vi "o3 Serial Comms Test.vi"() -> ()   [LabVIEW 2014]
uses:
  <vilib>/Platform/TimedLoop/XDataNode/timing_clust.ctl
  <vilib>/Platform/TimedLoop/XDataNode/nitl_modes.ctl
  <vilib>/Platform/TimedLoop/XDataNode/wakeup.ctl
  <vilib>/Utility/error.llb/whitespace.ctl
  <vilib>/Instr/_visa.llb/VISA Configure Serial Port (Instr).vi
  <vilib>/platform/TimedLoop/XDataNode/XDataNode.xnode
  <vilib>/Platform/TimedLoop/XDataNode/XDNodeRunTimeDep.lvlib
panel:
  in  "stop 2":bool
  out "Internal packet":string[](array[string])
  out "Data String":string
  out "Read Error Counter\nfrom process loop":i32
  out "Scan from String Error Counter\nfrom process loop":i32
  out "Data Array":string[](array[string])
  out "Data Processing":bool
  out "Serial Visa Error":errorcluster
  out "output 1":string
  out "error out 2":errorcluster
  out "Data In Array":string[](array[string])
  out "Number of Send & Read Error\nfrom Acquire Loop":i32
  out "Command In":string
  out "RAW DATA":string
  in  "ID 2":string="‚"
  in  "stop":bool
  in  "Command Input":string
  in  "VISA resource name 2":refnum<visa-resource-name>="ASRL6::INSTR"
  out "error out":errorcluster
  in  "Wait Time(mSec)":u32=330 caption="Count(mSec)"
  out "Loop counter":i32
  out "Max Acq Time":u32
  out "Write & Read Time (msec)":u32(graph)
  out "Running?":bool
  out "String":string
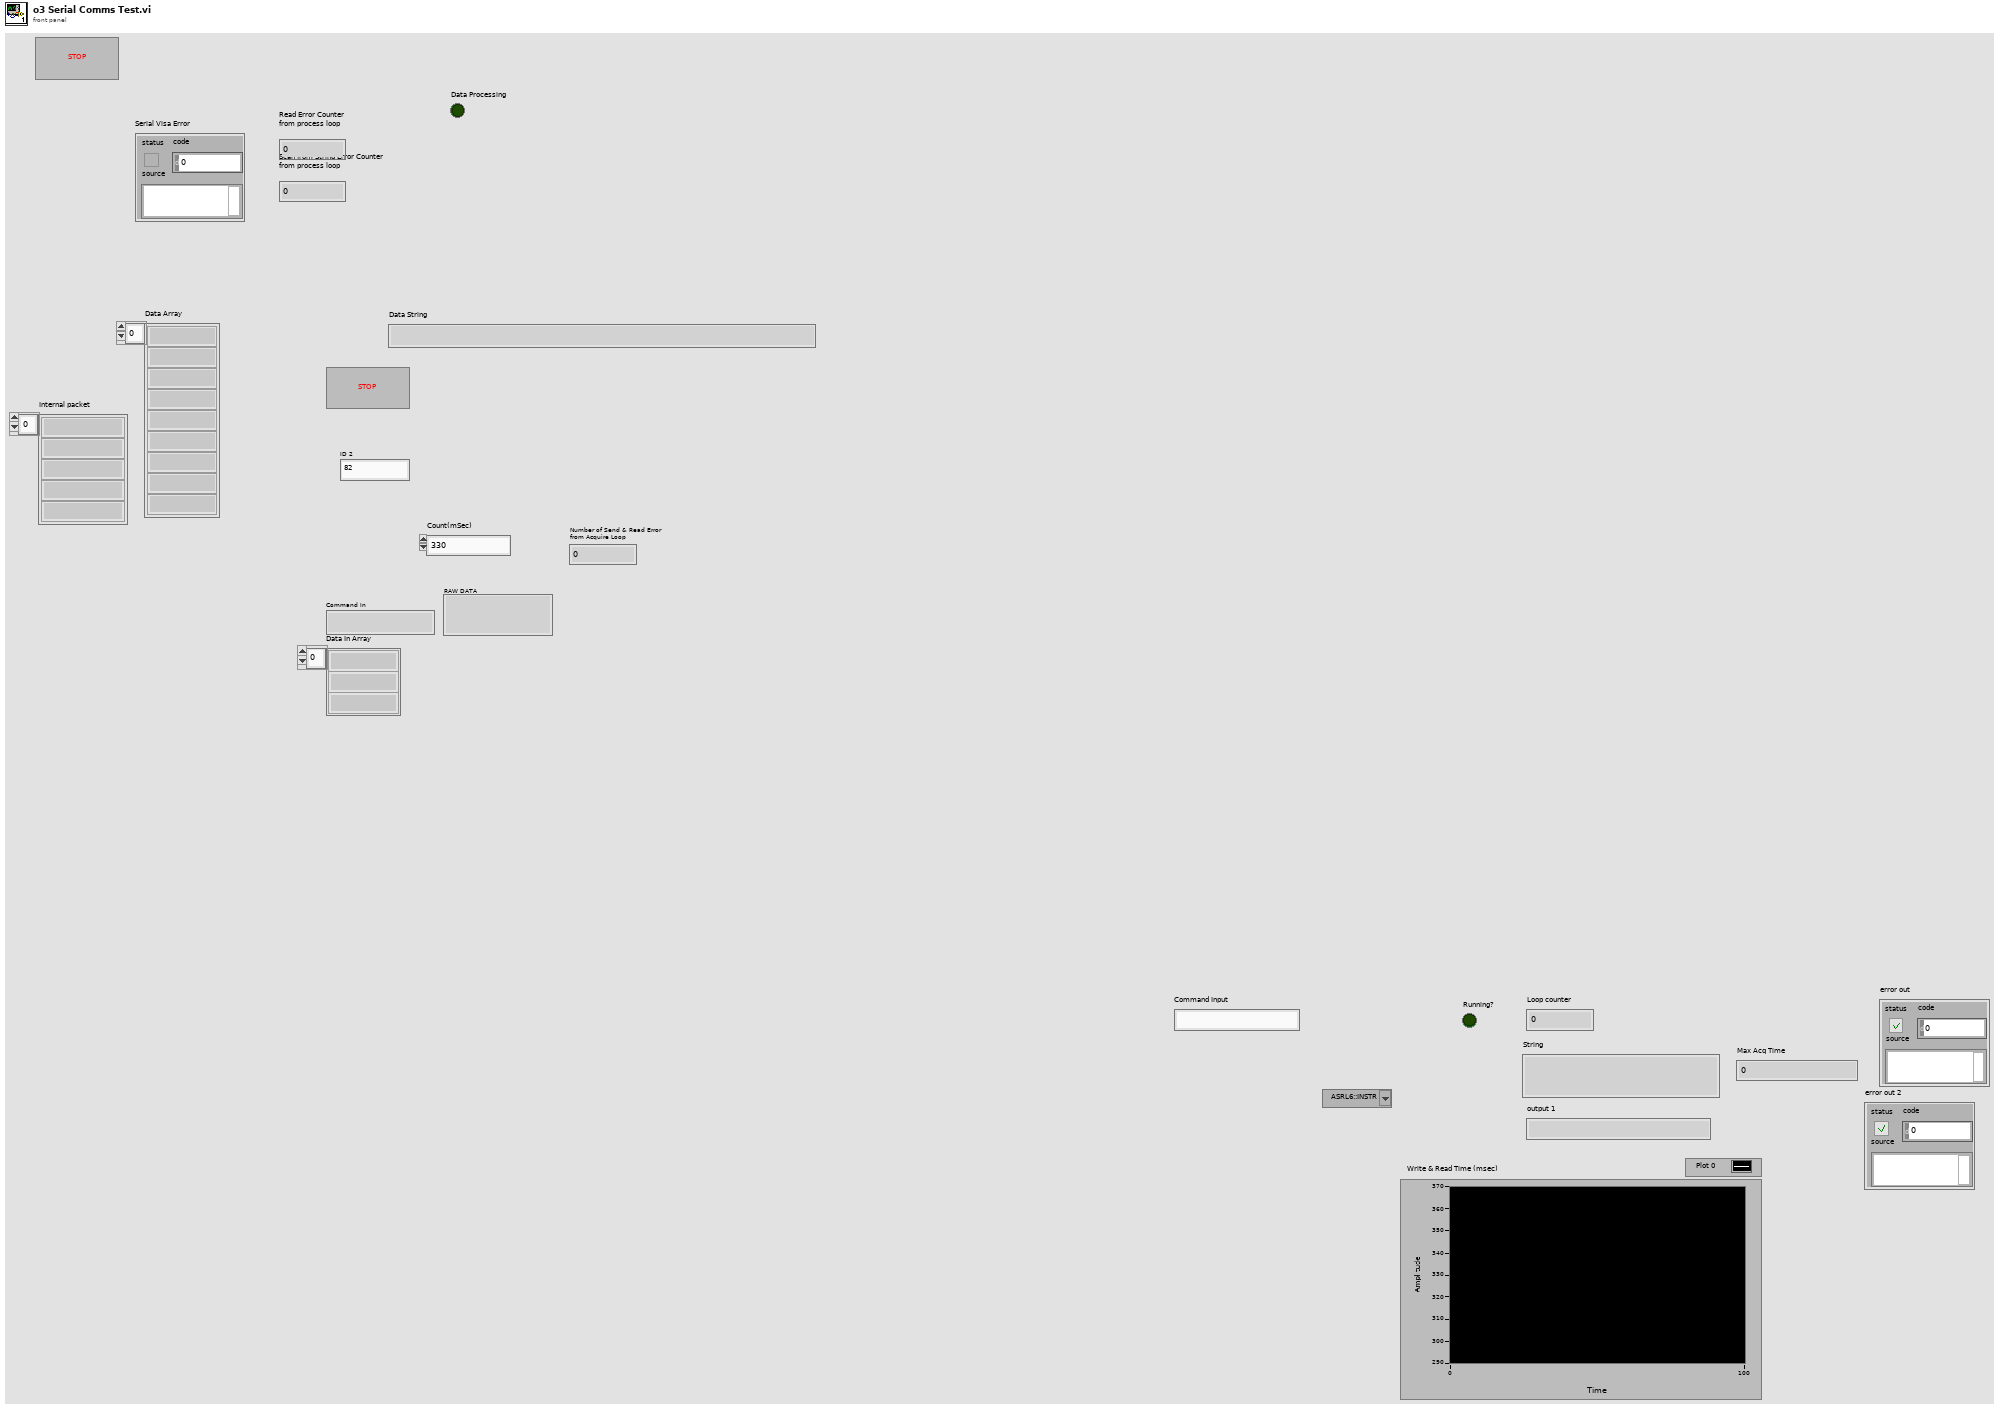
[diagram p1: front panel]
types:
  T1 = typedef "XDNodeRunTimeDep.lvlib/timing_clust.ctl" = cluster{"Expected End [f-1]":u64, "Actual End [f-1]":u64, "Finished Late? [f-1]":bool, "Expected End [i-1]":u64, "Actual End [i-1]":u64, "Finished Late? [i-1]":bool, "Expected Start [i]":u64, "Actual Start [i]":u64, "Expected Start [f]":u64, "Actual Start [f]":u64, "Source Name":string, "Structure Name":string, "Period":i64, "Deadline":i64, "Offset":i64, "Start":i64, "Priority":i32, "Timeout":i32, "Mode":T2, "Wakeup Reason":T3, "Error":errorcluster, "Source Type":string, "Secondary Source Type":string, "Global End Time":u64, "Global Start Time":u64, "Frame Duration":u64, "Iteration Duration":u64, "Assigned CPU":i32, "I/O Scan Engine Mode":u32}
  T2 = typedef "XDNodeRunTimeDep.lvlib/nitl_modes.ctl" = enum32{"No Change", "Process missed periods, maintain original phase", "Discard missed periods, maintain original phase", "Process missed periods, ignore original phase", "Discard missed periods, ignore original phase"}
  T3 = typedef "XDNodeRunTimeDep.lvlib/wakeup.ctl" = enum32{"Normal", "Aborted", "Asynchronous wakeup", "Timing source error", "Timed loop error", "Timeout"}
  T4 = typedef "whitespace.ctl" = u16
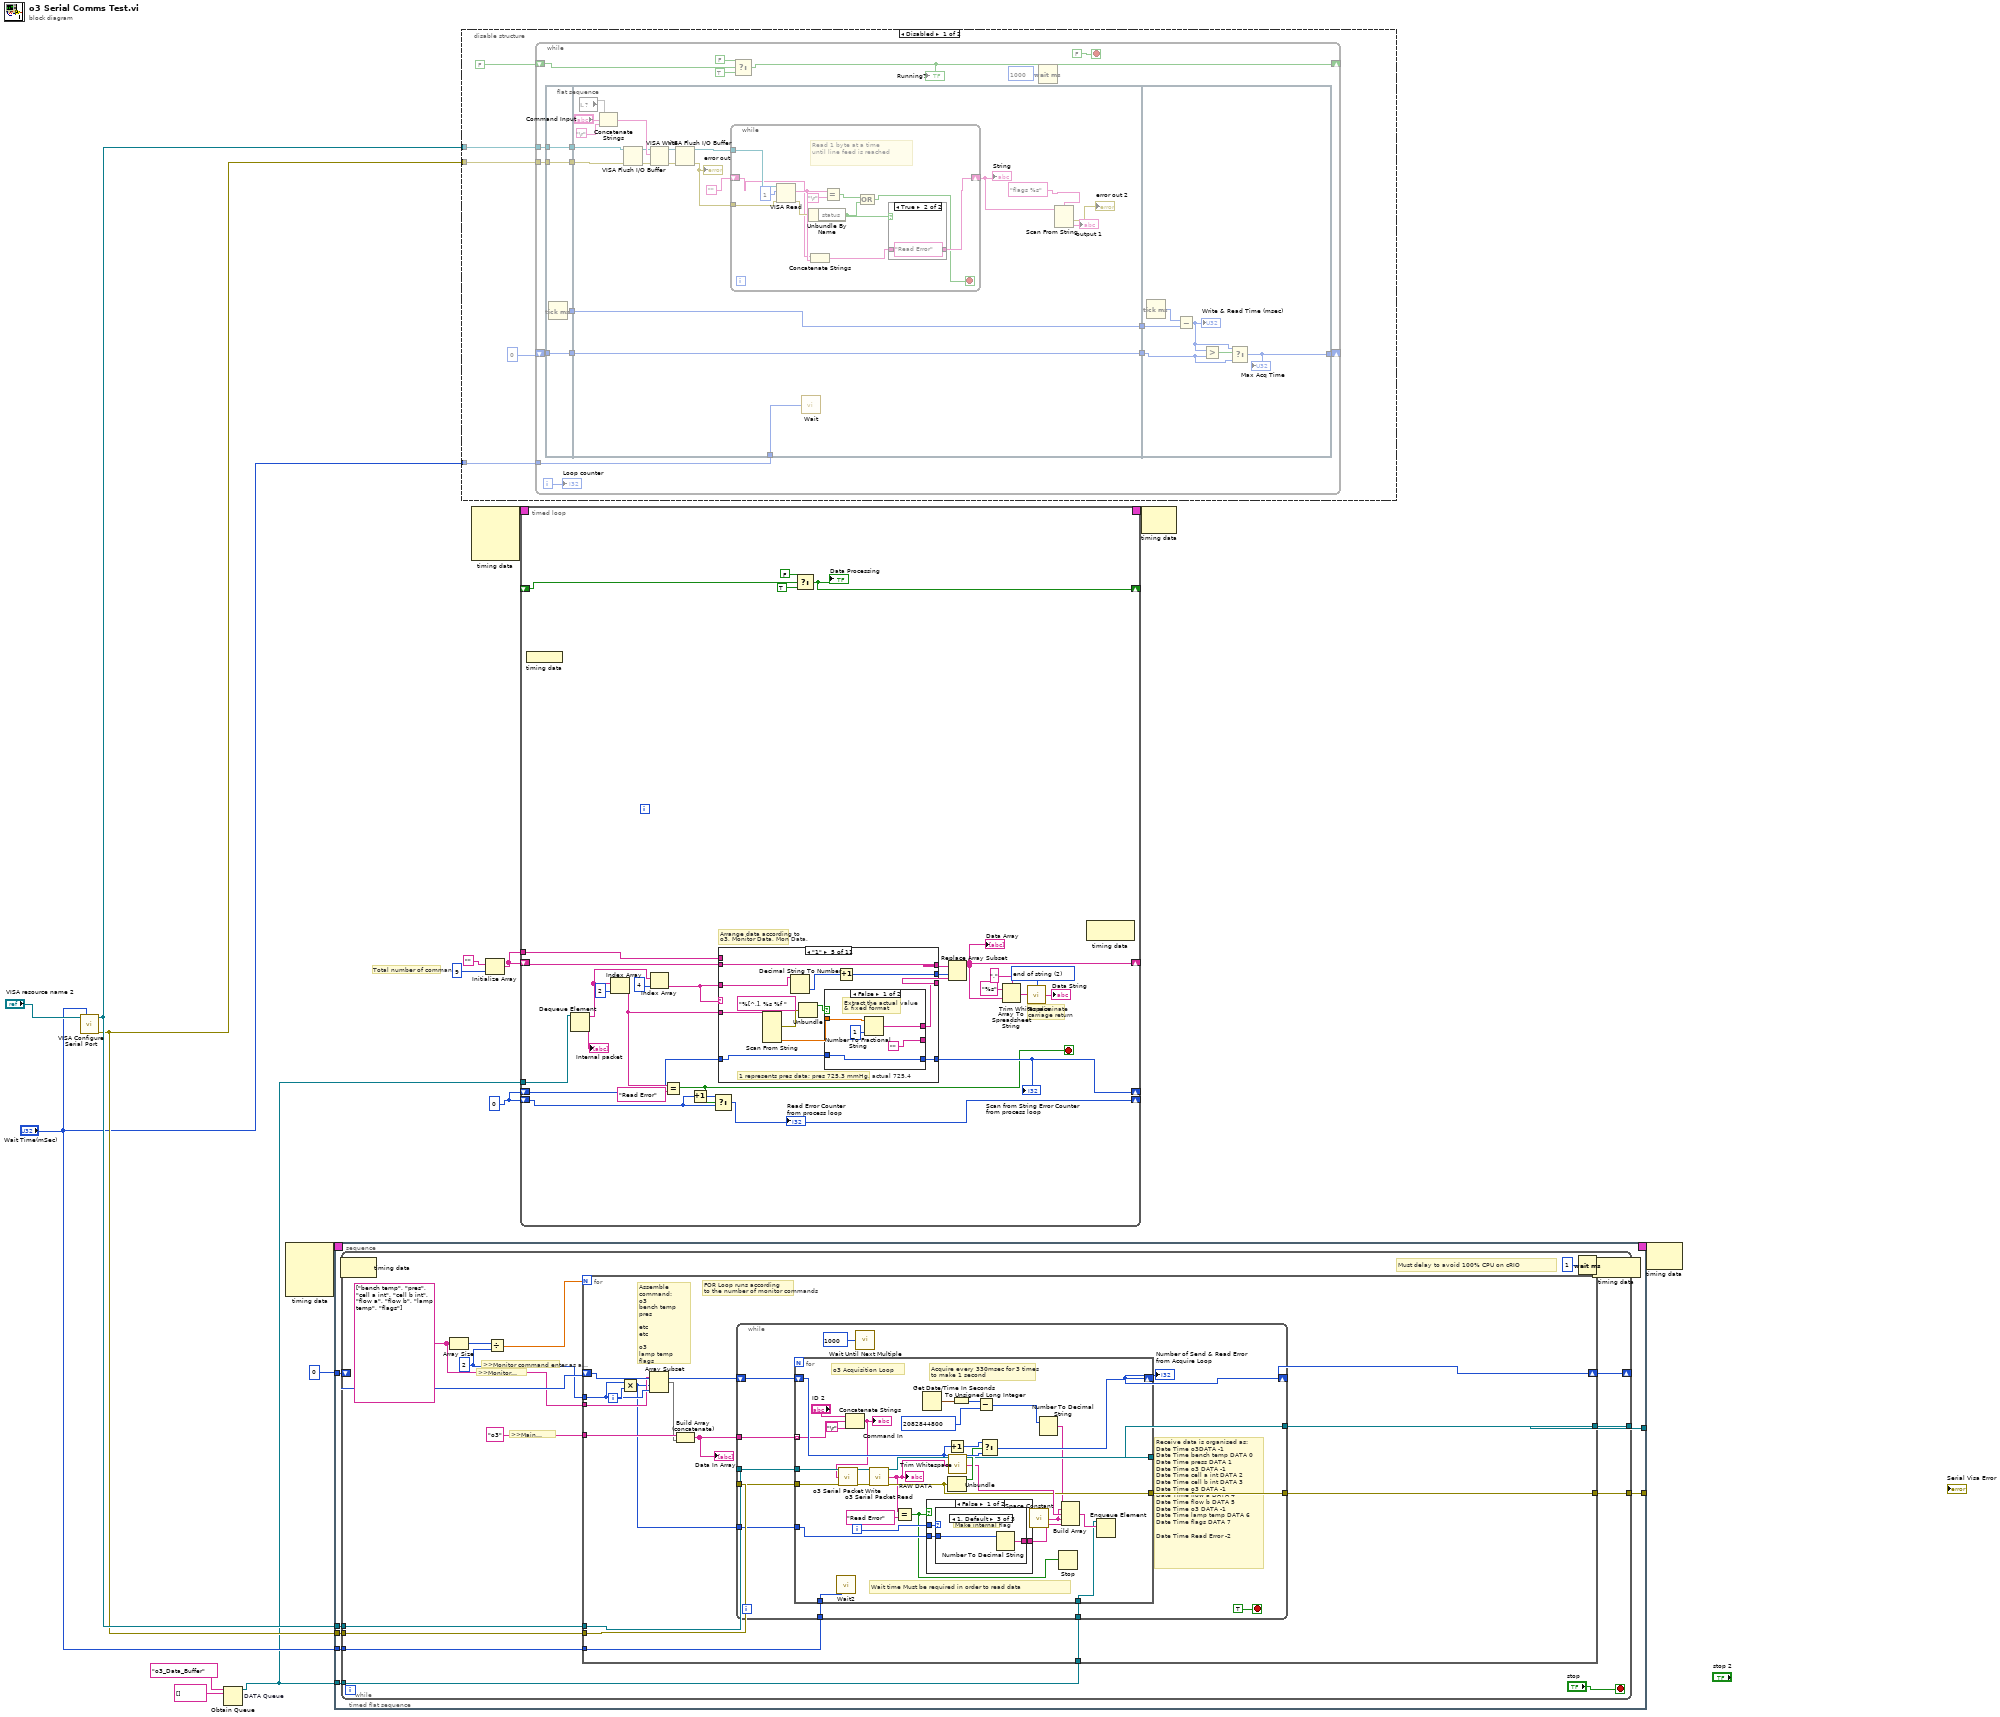
[diagram p0: block diagram]
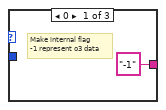
[diagram p2: hidden frame]
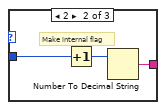
[diagram p3: hidden frame]
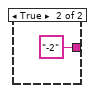
[diagram p4: hidden frame]
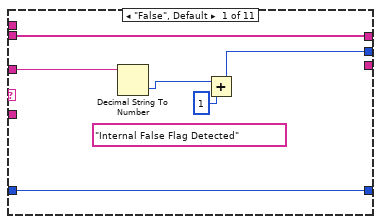
[diagram p7: hidden frame]
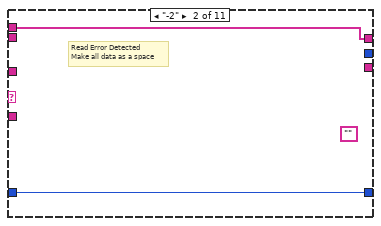
[diagram p8: hidden frame]
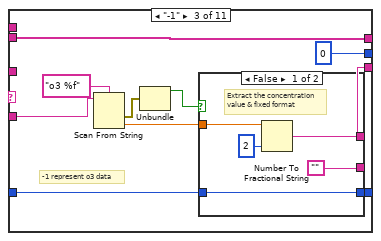
[diagram p9: hidden frame]
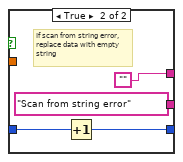
[diagram p10: hidden frame]
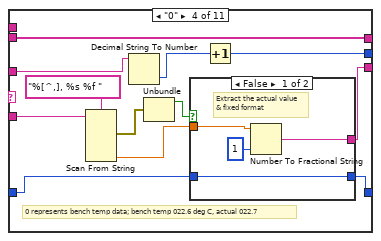
[diagram p11: hidden frame]
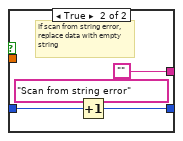
[diagram p12: hidden frame]
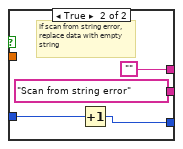
[diagram p13: hidden frame]
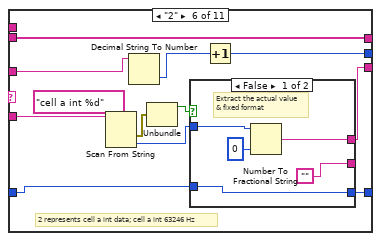
[diagram p14: hidden frame]
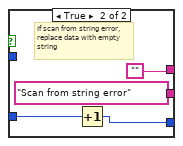
[diagram p15: hidden frame]
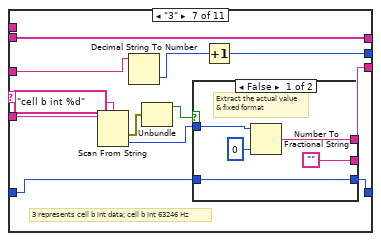
[diagram p16: hidden frame]
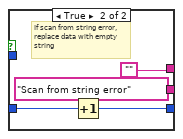
[diagram p17: hidden frame]
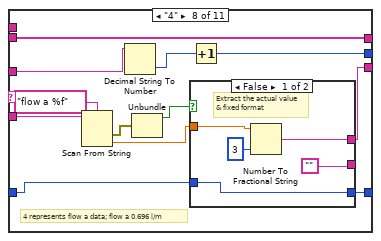
[diagram p18: hidden frame]
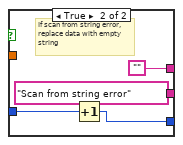
[diagram p19: hidden frame]
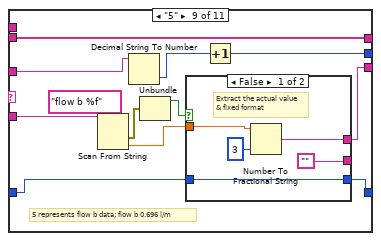
[diagram p20: hidden frame]
diagram:
  w4 = 0
  # "Total number of commands"
  n1 = call-poly "VISA Configure Serial Port"("VISA resource name"="VISA resource name 2", "timeout (10sec)"="Wait Time(mSec)") -> ("VISA resource name out"=w15:refnum<visa-resource-name>, "error out"=w14:errorcluster)  [unwired: 12 in]
  n2 = Obtain Queue "DATA Queue"(name (unnamed)="o3_Data_Buffer", element data type=string[] []) -> (queue out=w5:refnum<queue>)  [unwired: 3 in, 2 out]
  n3 = node-c288() -> (w8:T1)  [unwired: 4 in]
  n4 = timed-sequence {
    timing: w8 -> [_]
    timing-out: [_] -> w7
    tunnel: [w23] -> _
    tunnel: [w22] -> _
    tunnel: 0 -> [w21]
    tunnel: w14 -> [w20]
    tunnel: w15 -> [w19]
    tunnel: "Wait Time(mSec)" -> [w18]
    tunnel: w5 -> [w17]
    n5 = timed-flat-sequence {
      tunnel: [w30] -> w23
      tunnel: [w29] -> w22
      tunnel: w21 -> [w28]
      tunnel: w20 -> [w27]
      tunnel: w19 -> [w26]
      tunnel: w18 -> [w25]
      tunnel: w17 -> [w24]
      n6 = node-c288() -> ()  [unwired: 1 in, 1 out]
      n7 = while {
        tunnel: [w35] -> w30
        tunnel: w26 -> [w45]
        tunnel: w27 -> [w44]
        tunnel: [w43] -> w29
        shift-right: [w41] -> _
        shift-left: w28 -> [w42]
        tunnel: w25 -> [w33]
        tunnel: w24 -> [w31]
        stop <- "stop" stop-if-true
        w36 = 2
        w38 = string[] ["bench temp", "pres", "cell a int", "cell b int", "flow a", "flow b", "lamp temp", "flags"]
        # "Must delay to avoid 100% CPU on cRIO"
        # ">>Monitor command enter as a pair>>"
        # ">>Main commands>>"
        # ">>Monitor Command>>"
        n8 = Array Size(array=w38) -> (size(s)=w39:i32)
        n9 = Divide(x=w39, y=w36) -> (x/y=w37:dbl)
        n10 = for {
          N: w37 -> [_]
          tunnel: w45 -> [w54]
          tunnel: w44 -> [w53]
          tunnel: [w60] -> w35
          shift-right: [w58] -> w41
          shift-left: w42 -> [w59]
          tunnel: [w57] -> w43
          tunnel: w38 -> [w50]
          tunnel: "o3" -> [w55]
          tunnel: w36 -> [w51]
          tunnel: w33 -> [w47]
          tunnel: w31 -> [w46]
          i -> [w52]
          # "FOR Loop runs according\nto the number of monitor commands"
          # "Assemble command:\no3\nbench temp\npres\n\netc\netc\n\no3\nlamp temp\nflags"
          n11 = Multiply(x=w51, y=w52) -> (x*y=w48:i32)
          n12 = Array Subset(array=w50, index=w48, length=w51) -> (w49:string[])
          n13 = Build Array (concatenate)(w55, w49) -> (w56:string[])
          "Data In Array" <- w56
          n14 = while {
            tunnel: [w72] -> w60
            tunnel: w56 -> [w70]
            tunnel: [w68] -> w57
            tunnel: w53 -> [w67]
            tunnel: w54 -> [w66]
            tunnel: w48 -> [w65]
            shift-right: [w69] -> w58
            shift-left: w59 -> [w71]
            tunnel: w47 -> [w62]
            tunnel: w46 -> [w61]
            stop <- TRUE stop-if-true
            # "Receive data is organised as:\nDate Time o3DATA -1\nDate Time bench temp DATA 0\nDate Time press DATA 1\nDate Time o3 DATA -1\nDate Time cell a int DATA 2\nDate Time cell b int DATA 3\nDate Time o3 DATA -1\nDate Time flow a DATA 4\nDate Time flow b DATA 5\nDate Time o3 DATA -1\nDate Time lamp temp DATA 6\nDate Time flags DATA 7\n\nDate Time Read Error -2"
            n15 = for {
              tunnel: w67 -> [w90]
              tunnel: [w91] -> w72
              tunnel: w70 -> [w88] mode=indexing
              tunnel: [w92] -> w68
              tunnel: w66 -> [w93]
              tunnel: w65 -> [w87]
              shift-right: [w101] -> w69
              shift-left: w71 -> [w102]
              tunnel: w62 -> [w78]
              tunnel: w61 -> [w74]
              i -> [w82]
              # "Wait time Must be required in order to read data"
              # "Acquire every 330msec for 3 times\nto make 1 second"
              # "o3 Acquisition Loop"
              n16 = call "Wait2"("Count(mSec)"=w78) -> ()  [unwired: 1 out]
              n17 = Concatenate Strings("ID 2", w88, "\r") -> (w86:string)
              "Command In" <- w86
              n18 = call "o3 Serial Packet Write.vi"("VISA resource name In"=w93, "Data in"=w86, "error in (no error)"=w90) -> ("VISA resource name Out"=w95:refnum<visa-resource-name>, "error out"=w94:errorcluster)  [unwired: 11 in]
              n19 = call "o3 Serial Packet Read.vi"("VISA resource In"=w95, "error in"=w94) -> ("VISA resource Out"=w92:refnum<visa-resource-name>, "Data Out"=w84:string, "error out"=w91:errorcluster)  [unwired: 11 in]
              "RAW DATA" <- w84
              n20 = Equal?(x=w84, y="Read Error") -> (x = y?=w73:bool)
              n21 = Get Date/Time In Seconds() -> (seconds since 1Jan1904=w77:timestamp)
              n22 = case shown="False" w73 {
                tunnel: [w105 "-2"] -> w96
                tunnel: w82 -> [w104 _]
                tunnel: w87 -> [w103 _]
                frame False {
                  n23 = case shown="1, Default" w104 {
                    tunnel: ["-1" w109 w111] -> w105
                    tunnel: w103 -> [_ w107 w110]
                    frame 0 {
                      # "Make internal flag\n-1 represent o3 data"
                    }
                    frame 2 {
                      # "Make internal flag"
                      n24 = Increment(x=w107) -> (x+1=w108:i32)
                      n25 = Number To Decimal String(number=w108) -> (decimal integer string=w109:string)  [unwired: 1 in]
                    }
                    frame 1, Default {
                      # "Make internal flag"
                      n26 = Number To Decimal String(number=w110) -> (decimal integer string=w111:string)  [unwired: 1 in]
                    }
                  }
                }
                frame True {
                }
              }
              n27 = Increment(x=w102) -> (x+1=w98:i32)
              n28 = Unbundle(w91) -> ("status"=w99:bool)  [unwired: 2 out]
              n29 = call <vilib>:"Trim Whitespace.vi"("string"=w84) -> ("trimmed string"=w97:string)  [unwired: 1 in]
              n30 = To Unsigned Long Integer(number=w77) -> (unsigned 32bit integer=w81:u32)
              n31 = Subtract(x=w81, y=u32 2082844800) -> (x-y=w76:u32)
              n32 = Select(t=w98, s=w99, f=w102) -> (s? t:f=w101:i32)
              n33 = call <vilib>:"Space Constant.vi"() -> ("String"=w85:string)
              n34 = Number To Decimal String(number=w76) -> (decimal integer string=w79:string)  [unwired: 1 in]
              n35 = Stop(stop? (T)=w73) -> ()
              n36 = Build Array(w79, w85, w97, w85, w96) -> (w75:string[])
              n37 = Enqueue Element(queue=w74, element=w75) -> ()  [unwired: 2 in, 3 out]
            }
            "Number of Send & Read Error\nfrom Acquire Loop" <- w69
            n38 = call "Wait Until Next Multiple"("Count(mSec)"=u32 1000) -> ()  [unwired: 1 out]
          }
        }
        n39 = Wait (ms)(milliseconds to wait=u32 1) -> ()  [unwired: 1 out]
      }
      n40 = node-c288() -> ()  [unwired: 1 in, 1 out]
    }
  }
  n41 = disable-structure shown="Disabled" {
    disable-tunnel: w15 -> [w119 _]
    disable-tunnel: w14 -> [w118 _]
    disable-tunnel: "Wait Time(mSec)" -> [w117 _]
    frame Disabled {
      n42 = while {
        tunnel: w119 -> [w137]
        tunnel: w118 -> [w136]
        shift-right: [w131] -> _
        shift-left: FALSE -> [w134]
        shift-right: [w122] -> _
        shift-left: u32 0 -> [w124]
        tunnel: w117 -> [w120]
        i -> [w121]
        stop <- FALSE stop-if-true
        n43 = flat-sequence {
          tunnel: w136 -> [w140]
          tunnel: w137 -> [w141]
          tunnel: [w141] -> w129
          tunnel: [w140] -> w128
          tunnel: [w139] -> w127
          tunnel: [w138] -> w125
          tunnel: w124 -> [w138]
          tunnel: w129 -> [w155]
          tunnel: w128 -> [w154]
          tunnel: w127 -> [w149]
          tunnel: [w149] -> w126
          tunnel: w125 -> [w148]
          tunnel: [w148] -> w123
          tunnel: w120 -> [w147]
          tunnel: w126 -> [w180]
          tunnel: w123 -> [w177]
          tunnel: [w176] -> w122
          frame #0 {
            n44 = Tick Count (ms)() -> (millisecond timer value=w139:u32)
          }
          frame #1 {
            n45 = local read item#-1() -> (w161)
            n46 = Concatenate Strings(w161, "Command Input", "\r") -> (w157:string)
            n47 = VISA Flush I/O Buffer(VISA resource name=w155, error in (no error)=w154) -> (VISA resource name out=w156:refnum<visa-resource-name>, error out=w159:errorcluster)  [unwired: 1 in]
            n48 = VISA Write(VISA resource name=w156, write buffer=w157, error in (no error)=w159) -> (VISA resource name out=w153:refnum<visa-resource-name>, error out=w160:errorcluster)  [unwired: 1 out]
            n49 = VISA Flush I/O Buffer(VISA resource name=w153, error in (no error)=w160) -> (VISA resource name out=w151:refnum<visa-resource-name>, error out=w150:errorcluster)  [unwired: 1 in]
            "error out" <- w150
            n50 = while {
              shift-right: [w164] -> w144
              shift-left: "" -> [w165]
              tunnel: w151 -> [w166]
              tunnel: w150 -> [w162]
              stop <- w163 stop-if-true
              # "Read 1 byte at a time \nuntil line feed is reached"
              n51 = VISA Read(VISA resource name=w166, byte count=u32 1, error in (no error)=w162) -> (read buffer=w173:string, error out=w170:errorcluster)  [unwired: 2 out]
              n52 = Unbundle By Name(w170) -> ("status"=w168:bool)
              n53 = Concatenate Strings(w165, w173) -> (w169:string)
              n54 = Equal?(x=w173, y="\r") -> (x = y?=w167:bool)
              n55 = Compound Arithmetic op=OR(w167, w168) -> (w163:bool)
              n56 = case shown="True" w168 {
                tunnel: w169 -> [w174 _]
                tunnel: [w174 "Read Error"] -> w164
                frame False {
                }
                frame True {
                }
              }
            }
            "String" <- w144
            n57 = call "Wait"("Count(mSec)"=w147) -> ()  [unwired: 1 out]
            n58 = Scan From String(format string="flags %s", input string=w144) -> (error out=→"error out 2":errorcluster, output 1=→"output 1":string)  [unwired: 3 in, 2 out]
          }
          frame #2 {
            n59 = Tick Count (ms)() -> (millisecond timer value=w181:u32)
            n60 = Subtract(x=w181, y=w180) -> (x-y=w178:u32)
            "Write & Read Time (msec)" <- w178
            n61 = Greater?(x=w178, y=w177) -> (0:w179:bool)
            n62 = Select(t=w178, s=w179, f=w177) -> (s? t:f=w176:u32)
            "Max Acq Time" <- w176
          }
        }
        n63 = Select(t=FALSE, s=w134, f=TRUE) -> (s? t:f=w131:bool)
        "Running?" <- w131
        n64 = Wait (ms)(milliseconds to wait=u32 1000) -> ()  [unwired: 1 out]
        "Loop counter" <- w121
      }
    }
    frame Enabled {
    }
  }
  n65 = node-c288() -> (w12:T1)  [unwired: 4 in]
  n66 = Initialize Array("", 9) -> (w1:string[])
  n67 = timed-loop {
    timing: w12 -> [_]
    timing-out: [_] -> w11
    tunnel: w5 -> [w209]
    shift-right: [w189] -> _
    shift-left: w1 -> [w206]
    shift-right: [w195] -> _
    shift-left: w4 -> [w192]
    tunnel: w1 -> [w194]
    shift-right: [w190] -> _
    shift-left: w4 -> [w191]
    shift-right: [w184] -> _
    shift-left: _ -> [w186]
    stop <- w182 stop-if-true
    w199 = T4 2 items=["both", "start of string", "end of string"] ("location (both)")
    # "Arrange data according to\no3, Monitor Data, Mon Data,"
    # "To eliminate\ncarriage return"
    n68 = node-c288() -> ()  [unwired: 1 in]
    n69 = Dequeue Element(queue=w209) -> (element=w187:string[])  [unwired: 2 in, 3 out]
    "Internal packet" <- w187
    n70 = Index Array(array=w187, index=2) -> (element=w197:string)
    n71 = Index Array(array=w187, index=4) -> (element=w205:string)
    n72 = Equal?(x=w197, y="Read Error") -> (x = y?=w182:bool)
    n73 = Increment(x=w192) -> (x+1=w193:i32)
    n74 = Select(t=w193, s=w182, f=w192) -> (s? t:f=w195:i32)
    "Read Error Counter\nfrom process loop" <- w195
    n75 = case shown="\"1\"" w205 {
      tunnel: w205 -> [w214 _ _ w247 w266 w287 w308 w329 w350 w371 w392]
      tunnel: w206 -> [w215 _ w227 w248 w267 w288 w309 w330 w351 w372 w393]
      tunnel: w197 -> [_ _ w224 w243 w262 w284 w305 w326 w347 w368 w389]
      tunnel: [w215 w217 w227 w248 w267 w288 w309 w330 w351 w372 w393] -> w204
      tunnel: [w212 _ 0 ("index") w245 w264 w285 w306 w327 w348 w369 w390] -> w203
      tunnel: [_ _ w222 w241 w260 w283 w304 w325 w346 w367 w384] -> w202
      tunnel: w194 -> [_ w217 _ _ _ _ _ _ _ _ _]
      tunnel: w191 -> [w210 w216 w219 w238 w257 w278 w299 w320 w341 w362 w383]
      tunnel: [w210 w216 w218 w237 w256 w277 w298 w319 w340 w361 w382] -> w190
      frame "False", Default {
        (unwired) "Internal False Flag Detected"
        n76 = Decimal String To Number(string=w214) -> (number=w211:i32)  [unwired: 2 in, 1 out]
        n77 = Add(x=w211, y=1) -> (x+y=w212:i32)
      }
      frame "-2" {
        (unwired) ""
        # "Read Error Detected\nMake all data as a space"
      }
      frame "-1" {
        # "-1 represent o3 data"
        n78 = Scan From String(format string="o3 %f", input string=w224) -> (error out=w221:errorcluster, output 1=w223:dbl)  [unwired: 3 in, 2 out]
        n79 = Unbundle(w221) -> ("status"=w220:bool)  [unwired: 2 out]
        n80 = case shown="False" w220 {
          tunnel: w223 -> [w232 _]
          tunnel: [w231 ""] -> w222
          tunnel: w219 -> [w230 w235]
          tunnel: [w230 w234] -> w218
          tunnel: ["" "Scan from string error"] -> _
          frame False {
            # "Extract the concentration\nvalue & fixed format"
            n81 = Number To Fractional String(number=w232, precision (6)=i16 2) -> (F-format string=w231:string)  [unwired: 2 in]
          }
          frame True {
            # "If scan from string error,\nreplace data with empty\nstring"
            n82 = Increment(x=w235) -> (x+1=w234:i32)
          }
        }
      }
      frame "0" {
        # "0 represents bench temp data; bench temp 022.6 deg C, actual 022.7"
        n83 = Scan From String(format string="%[^,], %s %f ", input string=w243) -> (error out=w240:errorcluster, output 3=w242:dbl)  [unwired: 7 in, 2 out]
        n84 = Decimal String To Number(string=w247) -> (number=w246:i32)  [unwired: 2 in, 1 out]
        n85 = Unbundle(w240) -> ("status"=w239:bool)  [unwired: 2 out]
        n86 = case shown="False" w239 {
          tunnel: w242 -> [w252 _]
          tunnel: [w251 ""] -> w241
          tunnel: w238 -> [w250 w254]
          tunnel: [w250 w253] -> w237
          frame False {
            # "Extract the actual value\n& fixed format"
            n87 = Number To Fractional String(number=w252, precision (6)=i16 1) -> (F-format string=w251:string)  [unwired: 2 in]
          }
          frame True {
            (unwired) "Scan from string error"
            # "If scan from string error,\nreplace data with empty\nstring"
            n88 = Increment(x=w254) -> (x+1=w253:i32)
          }
        }
        n89 = Increment(x=w246) -> (x+1=w245:i32)
      }
      frame "1" {
        # "1 represents pres data; pres 725.3 mmHg, actual 725.4"
        n90 = Scan From String(format string="%[^,], %s %f ", input string=w262) -> (error out=w259:errorcluster, output 3=w261:dbl)  [unwired: 7 in, 2 out]
        n91 = Decimal String To Number(string=w266) -> (number=w265:i32)  [unwired: 2 in, 1 out]
        n92 = Unbundle(w259) -> ("status"=w258:bool)  [unwired: 2 out]
        n93 = case shown="False" w258 {
          tunnel: w261 -> [w272 _]
          tunnel: [w271 ""] -> w260
          tunnel: w257 -> [w270 w275]
          tunnel: [w270 w274] -> w256
          tunnel: ["" "Scan from string error"] -> _
          frame False {
            # "Extract the actual value\n& fixed format"
            n94 = Number To Fractional String(number=w272, precision (6)=i16 1) -> (F-format string=w271:string)  [unwired: 2 in]
          }
          frame True {
            # "If scan from string error,\nreplace data with empty\nstring"
            n95 = Increment(x=w275) -> (x+1=w274:i32)
          }
        }
        n96 = Increment(x=w265) -> (x+1=w264:i32)
      }
      frame "2" {
        # "2 represents cell a int data; cell a int 63246 Hz"
        n97 = Scan From String(format string="cell a int %d", input string=w284) -> (error out=w280:errorcluster, output 1=w281:i32)  [unwired: 3 in, 2 out]
        n98 = Decimal String To Number(string=w287) -> (number=w286:i32)  [unwired: 2 in, 1 out]
        n99 = Unbundle(w280) -> ("status"=w279:bool)  [unwired: 2 out]
        n100 = case shown="False" w279 {
          tunnel: [w293 ""] -> w283
          tunnel: w281 -> [w292 _]
          tunnel: w278 -> [w291 w296]
          tunnel: [w291 w295] -> w277
          tunnel: ["" "Scan from string error"] -> _
          frame False {
            # "Extract the actual value\n& fixed format"
            n101 = Number To Fractional String(number=w292, precision (6)=i16 0) -> (F-format string=w293:string)  [unwired: 2 in]
          }
          frame True {
            # "If scan from string error,\nreplace data with empty\nstring"
            n102 = Increment(x=w296) -> (x+1=w295:i32)
          }
        }
        n103 = Increment(x=w286) -> (x+1=w285:i32)
      }
      frame "3" {
        # "3 represents cell b int data; cell b int 63246 Hz"
        n104 = Scan From String(format string="cell b int %d", input string=w305) -> (error out=w301:errorcluster, output 1=w302:i32)  [unwired: 3 in, 2 out]
        n105 = Decimal String To Number(string=w308) -> (number=w307:i32)  [unwired: 2 in, 1 out]
        n106 = Unbundle(w301) -> ("status"=w300:bool)  [unwired: 2 out]
        n107 = case shown="False" w300 {
          tunnel: [w314 ""] -> w304
          tunnel: w302 -> [w313 _]
          tunnel: w299 -> [w312 w317]
          tunnel: [w312 w316] -> w298
          tunnel: ["" "Scan from string error"] -> _
          frame False {
            # "Extract the actual value\n& fixed format"
            n108 = Number To Fractional String(number=w313, precision (6)=i16 0) -> (F-format string=w314:string)  [unwired: 2 in]
          }
          frame True {
            # "If scan from string error,\nreplace data with empty\nstring"
            n109 = Increment(x=w317) -> (x+1=w316:i32)
          }
        }
        n110 = Increment(x=w307) -> (x+1=w306:i32)
      }
      frame "4" {
        # "4 represents flow a data; flow a 0.696 l/m"
        n111 = Scan From String(format string="flow a %f", input string=w326) -> (error out=w322:errorcluster, output 1=w323:dbl)  [unwired: 3 in, 2 out]
        n112 = Decimal String To Number(string=w329) -> (number=w328:i32)  [unwired: 2 in, 1 out]
        n113 = Unbundle(w322) -> ("status"=w321:bool)  [unwired: 2 out]
        n114 = case shown="False" w321 {
          tunnel: [w335 ""] -> w325
          tunnel: w323 -> [w334 _]
          tunnel: w320 -> [w333 w338]
          tunnel: [w333 w337] -> w319
          tunnel: ["" "Scan from string error"] -> _
          frame False {
            # "Extract the actual value\n& fixed format"
            n115 = Number To Fractional String(number=w334, precision (6)=i16 3) -> (F-format string=w335:string)  [unwired: 2 in]
          }
          frame True {
            # "If scan from string error,\nreplace data with empty\nstring"
            n116 = Increment(x=w338) -> (x+1=w337:i32)
          }
        }
        n117 = Increment(x=w328) -> (x+1=w327:i32)
      }
      frame "5" {
        # "5 represents flow b data; flow b 0.696 l/m"
        n118 = Scan From String(format string="flow b %f", input string=w347) -> (error out=w343:errorcluster, output 1=w344:dbl)  [unwired: 3 in, 2 out]
        n119 = Decimal String To Number(string=w350) -> (number=w349:i32)  [unwired: 2 in, 1 out]
        n120 = Unbundle(w343) -> ("status"=w342:bool)  [unwired: 2 out]
        n121 = case shown="False" w342 {
          tunnel: [w356 ""] -> w346
          tunnel: w344 -> [w355 _]
          tunnel: w341 -> [w354 w359]
          tunnel: [w354 w358] -> w340
          tunnel: ["" "Scan from string error"] -> _
          frame False {
            # "Extract the actual value\n& fixed format"
            n122 = Number To Fractional String(number=w355, precision (6)=i16 3) -> (F-format string=w356:string)  [unwired: 2 in]
          }
          frame True {
            # "If scan from string error,\nreplace data with empty\nstring"
            n123 = Increment(x=w359) -> (x+1=w358:i32)
          }
        }
        n124 = Increment(x=w349) -> (x+1=w348:i32)
      }
      frame "6" {
        # "6 represents lamp temp data; lamp temp 056.1 deg C"
        n125 = Scan From String(format string="lamp temp %f", input string=w368) -> (error out=w364:errorcluster, output 1=w365:dbl)  [unwired: 3 in, 2 out]
        n126 = Decimal String To Number(string=w371) -> (number=w370:i32)  [unwired: 2 in, 1 out]
        n127 = Unbundle(w364) -> ("status"=w363:bool)  [unwired: 2 out]
        n128 = case shown="False" w363 {
          tunnel: [w377 ""] -> w367
          tunnel: w365 -> [w376 _]
          tunnel: w362 -> [w375 w380]
          tunnel: [w375 w379] -> w361
          tunnel: ["" "Scan from string error"] -> _
          frame False {
            # "Extract the actual value\n& fixed format"
            n129 = Number To Fractional String(number=w376, precision (6)=i16 1) -> (F-format string=w377:string)  [unwired: 2 in]
          }
          frame True {
            # "If scan from string error,\nreplace data with empty\nstring"
            n130 = Increment(x=w380) -> (x+1=w379:i32)
          }
        }
        n131 = Increment(x=w370) -> (x+1=w369:i32)
      }
      frame "7" {
        # "7 represents flags data; flags 1c100000"
        n132 = Scan From String(format string="flags %s", input string=w389) -> (error out=w387:errorcluster, output 1=w385:string)  [unwired: 3 in, 2 out]
        n133 = Decimal String To Number(string=w392) -> (number=w391:i32)  [unwired: 2 in, 1 out]
        n134 = Unbundle(w387) -> ("status"=w386:bool)  [unwired: 2 out]
        n135 = case shown="False" w386 {
          tunnel: w385 -> [w396 _]
          tunnel: [w396 ""] -> w384
          tunnel: w383 -> [w395 w399]
          tunnel: [w395 w398] -> w382
          tunnel: ["" "Scan from string error"] -> _
          frame False {
            # "Extract the actual value\n& fixed format"
          }
          frame True {
            # "If scan from string error,\nreplace data with empty\nstring"
            n136 = Increment(x=w399) -> (x+1=w398:i32)
          }
        }
        n137 = Increment(x=w391) -> (x+1=w390:i32)
      }
    }
    "Scan from String Error Counter\nfrom process loop" <- w190
    n138 = Select(t=FALSE, s=w186, f=TRUE) -> (s? t:f=w184:bool)
    "Data Processing" <- w184
    n139 = Replace Array Subset(array=w204, new element=w202, index=w203) -> (w189:string[])
    "Data Array" <- w189
    n140 = Array To Spreadsheet String(delimiter (Tab)=",", array=w189, 3:"%s" ("format string")) -> (spreadsheet string=w198:string)
    n141 = call <vilib>:"Trim Whitespace.vi"("string"=w198, "location (both)"=w199) -> ("trimmed string"=→"Data String":string)
    n142 = node-c288() -> ()  [unwired: 1 in, 1 out]
  }
  n143 = node-c288(w11) -> ()  [unwired: 1 out]
  n144 = node-c288(w7) -> ()  [unwired: 1 out]
